vi "ShooterWhileLoop.vi"(11 "Boolean":bool) -> ()   [LabVIEW 2012]
uses:
  Robot Global Data.vi
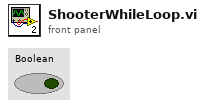
[diagram p1: front panel]
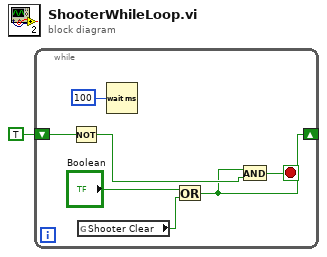
[diagram p0: block diagram]
diagram:
  n1 = while {
    shift-right: [w2] -> _
    shift-left: TRUE -> [w7]
    stop <- w6 stop-if-true
    n2 = Not(x=w7) -> (.not. x?=w3:bool)
    n3 = global read "Robot Global Data.vi" "Shooter Clear"() -> (w5:bool)
    n4 = Wait (ms)(milliseconds to wait=u32 100 ("millisecond timer value")) -> ()  [unwired: 1 out]
    n5 = Or(x="Boolean", y=w5) -> (x .or. y?=w2:bool)
    n6 = And(x=w2, y=w3) -> (x .and. y?=w6:bool)
  }
